vi "Fill Slider Values.vi"(10 "LBCB Number":T3, 11 "DofType":T2) -> (2 "Silder Values":T1(array[cluster]))   [LabVIEW 2009]
uses:
  Data Access Objects/Metadata/LBCB Number.ctl
  Data Access Objects/Limits/DofTypes.ctl
  Data Access Objects/Metadata/Persistant DAO Actions.ctl
  Global Data/Dataset Type.ctl
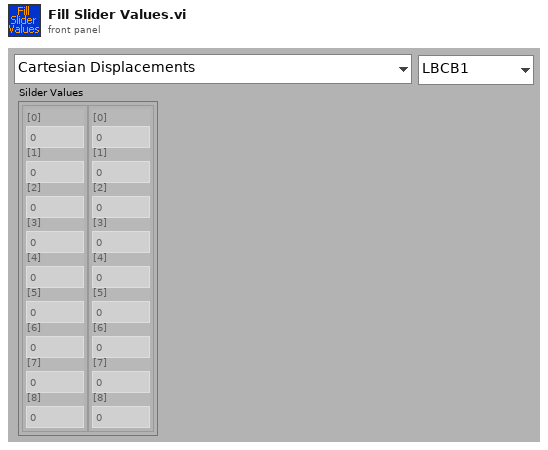
[diagram p1: front panel]
types:
  T1 = cluster{"[0]":dbl, "[1]":dbl, "[2]":dbl, "[3]":dbl, "[4]":dbl, "[5]":dbl, "[6]":dbl, "[7]":dbl, "[8]":dbl}[]
  T2 = typedef "DofTypes.ctl" = enum16{"Cartesian Displacements", "Cartesian Forces & Moments", "Actuator Displacements", "Actuator Forces", "Cartesian Increments", "Actuator Increments"}
  T3 = typedef "LBCB Number.ctl" = enum16{"LBCB1", "LBCB2"}
  T4 = typedef "Dataset Type.ctl" = enum16{"LVDT", "Load Cell", "Actuator Command", "Servo Error", "Displacement Command", "Displacement", "Force"}
  T5 = typedef "Persistant DAO Actions.ctl" = enum16{"Init", "Get", "Set", "Load", "Save"}
  T6 = typedef "Dataset Source.ctl" = enum16{"LBCB 1", "LBCB 2", "Combined", "External Sensors"}
  T7 = typedef "Dataset Transaction Id.ctl" = cluster{"Dataset Source":T6, "Dataset Type":T4, "Hold":T8, "Volts":T8, "Tag":string}
  T8 = typedef "Yes No Button.ctl" = bool
  T9 = typedef "Actuator Matrix.ctl" = cluster{"Lower":T10, "Upper":T10}
  T10 = typedef "Actuator Point.ctl" = cluster{"X1":dbl, "X2":dbl, "Y1":dbl, "Z1":dbl, "Z2":dbl, "Z3":dbl}
  T11 = typedef "Cartesian Point.ctl" = cluster{"Dx":dbl, "Dy":dbl, "Dz":dbl, "Rx":dbl, "Ry":dbl, "Rz":dbl}
  T12 = typedef "Cartesian Matrix.ctl" = cluster{"Lower":T11, "Upper":T11}
  T13 = typedef "Act & Cart Commands.ctl" = cluster{"Act Cmd":dbl[], "Cart Cmd":dbl[]}
  T14 = typedef "Limit Matrix.ctl" = dbl[][]
  T15 = cluster{"[0]":dbl, "[1]":dbl, "[2]":dbl, "[3]":dbl, "[4]":dbl, "[5]":dbl, "[6]":dbl, "[7]":dbl, "[8]":dbl}[][]
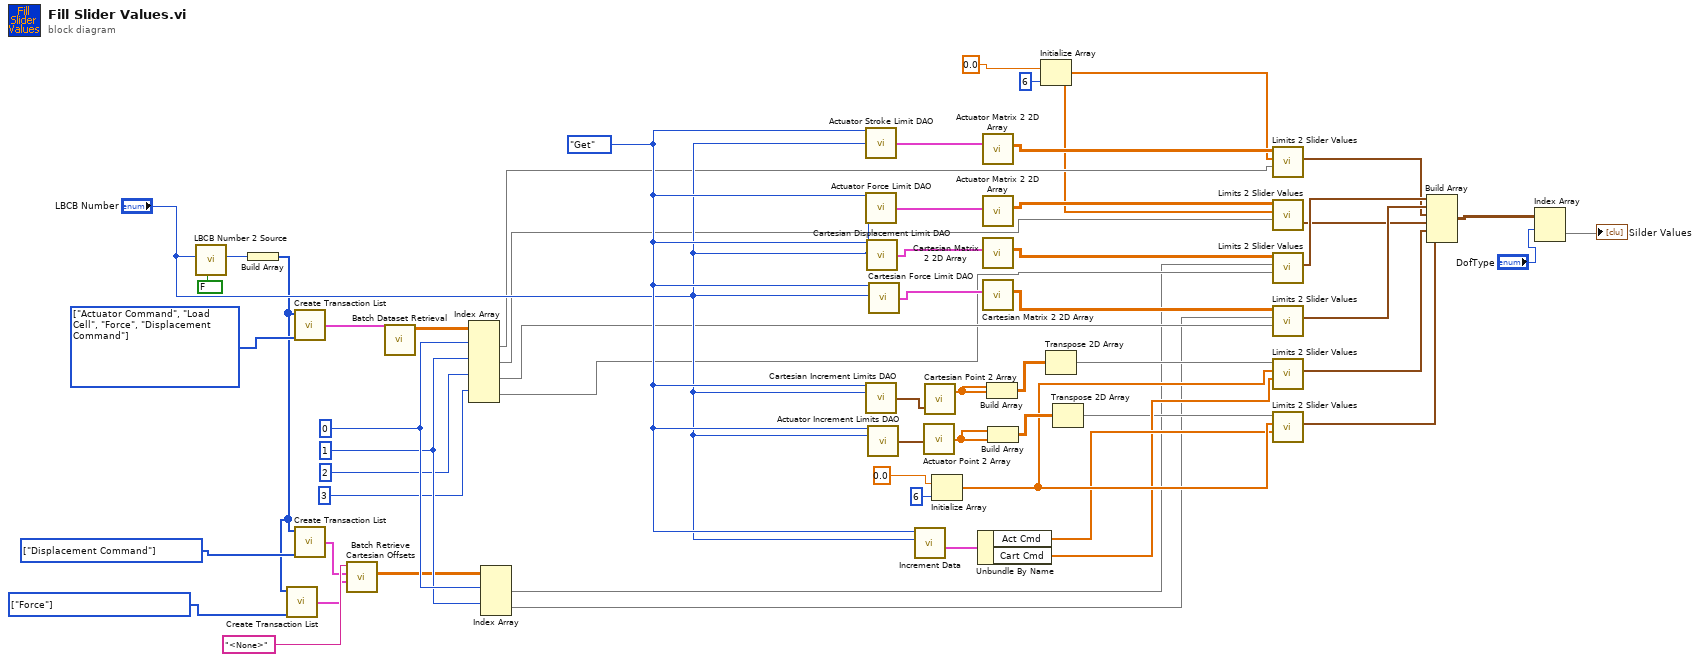
[diagram p0: block diagram]
diagram:
  w9 = T4[] [enum."Force"] items=["LVDT", "Load Cell", "Actuator Command", "Servo Error", "Displacement Command", "Displacement", "Force"] ("Types")
  w10 = T4[] [enum."Displacement Command"] items=["LVDT", "Load Cell", "Actuator Command", "Servo Error", "Displacement Command", "Displacement", "Force"] ("Types")
  w16 = 1 ("index")
  w17 = 0 ("index (row)")
  w26 = T4[] [enum."Actuator Command", enum."Load Cell", enum."Force", enum."Displacement Command"] items=["LVDT", "Load Cell", "Actuator Command", "Servo Error", "Displacement Command", "Displacement", "Force"] ("Types")
  w34 = Persistant_DAO_Actions."Get" ("Actuator Stroke Limit Actions")
  n1 = call "LBCB Number 2 Source.vi"("Combined"=FALSE, "LBCB Number"="LBCB Number") -> ("Dataset Source"=w25:T6)  [unwired: 9 in]
  n2 = Build Array(w25) -> (w8:T6[])
  n3 = call "Create Transaction List.vi"("Types"=w9, "Sources"=w8) -> ("Transactions"=w5:T7[])  [unwired: 2 in]
  n4 = call "Create Transaction List.vi"("Types"=w26, "Sources"=w8) -> ("Transactions"=w23:T7[])  [unwired: 2 in]
  n5 = call "Create Transaction List.vi"("Types"=w10, "Sources"=w8) -> ("Transactions"=w6:T7[])  [unwired: 2 in]
  n6 = call "Batch Retrieve Cartesian Offsets.vi"("Force Offsets"=w5, "Displacement Offsets"=w6, "Force Tag"="<None>") -> ("Offsets"=w4:dbl[][])  [unwired: 5 in, 1 out]
  n7 = call "Batch Dataset Retrieval.vi"("Transactions"=w23) -> ("Data"=w22:dbl[][])  [unwired: 9 in, 1 out]
  n8 = Index Array(array=w22, index (row) #1=w17, index (row) #2=w16, index (row) #3=2 ("index"), index (row) #4=3 ("index")) -> (element #1=w21:dbl[], element #2=w20:dbl[], element #3=w19:dbl[], element #4=w18:dbl[])  [unwired: 4 in]
  n9 = Index Array(array=w4, index (row) #1=w17, index (row) #2=w16) -> (element #1=w3:dbl[], element #2=w2:dbl[])  [unwired: 2 in]
  n10 = call "Actuator Stroke Limit DAO.vi"("Actuator Stroke Limit Actions"=w34, "ID"="LBCB Number") -> ("Actuator Stroke Limits Out"=w58:T9)  [unwired: 11 in, 2 out]
  n11 = call "Actuator Force Limit DAO.vi"("Actuator Force Limit Actions"=w34, "ID"="LBCB Number") -> ("Actuator Force Limits Out"=w57:T9)  [unwired: 11 in, 2 out]
  n12 = call "Cartesian Increment Limits DAO.vi"("Actions"=w34, "LBCB Number"="LBCB Number") -> ("Inc Limits Out"=w43:T11)  [unwired: 11 in, 2 out]
  n13 = call "Cartesian Displacement Limit DAO.vi"("Cartesian Displacement Limit Actions"=w34, "ID"="LBCB Number") -> ("Cartesian Displacement Out"=w56:T12)  [unwired: 11 in, 2 out]
  n14 = call "Actuator Increment Limits DAO.vi"("Actions"=w34, "LBCB Number"="LBCB Number") -> ("Inc Limits Out"=w42:T10)  [unwired: 11 in, 2 out]
  n15 = call "Cartesian Force Limit DAO.vi"("Cartesian Force Limit Actions"=w34, "ID"="LBCB Number") -> ("Cartesian Force Limit Out"=w55:T12)  [unwired: 11 in, 2 out]
  n16 = call "Increment Data.vi"("LBCB Number"="LBCB Number", "DAO Actions"=w34) -> ("Increments Out"=w33:T13)  [unwired: 8 in, 1 out]
  n17 = call "Actuator Point 2 Array.vi"("Actuator Point"=w42) -> ("Array"=w40:dbl[])
  n18 = call "Cartesian Point 2 Array.vi"("Cart Disp"=w43) -> ("Array"=w41:dbl[])  [unwired: 2 in]
  n19 = Initialize Array(0.0 ("element"), 6 ("dimension size")) -> (w35:dbl[])
  n20 = Unbundle By Name(w33) -> ("Act Cmd"=w32:dbl[], "Cart Cmd"=w31:dbl[])
  n21 = call "Actuator Matrix 2 2D Array.vi"("Matrix In"=w58) -> ("Matrix Out"=w54:T14)  [unwired: 10 in]
  n22 = call "Actuator Matrix 2 2D Array.vi"("Matrix In"=w57) -> ("Matrix Out"=w53:T14)  [unwired: 10 in]
  n23 = call "Cartesian Matrix 2 2D Array.vi"("Matrix In"=w56) -> ("Matrix Out"=w52:T14)  [unwired: 10 in]
  n24 = call "Cartesian Matrix 2 2D Array.vi"("Matrix In"=w55) -> ("Matrix Out"=w51:T14)  [unwired: 10 in]
  n25 = Build Array(w41, w41) -> (w39:dbl[][])
  n26 = Build Array(w40, w40) -> (w38:dbl[][])
  n27 = Initialize Array(0.0, 6 ("dimension size")) -> (w11:dbl[])
  n28 = Transpose 2D Array(2D array=w39) -> (transposed array=w28:dbl[][])
  n29 = Transpose 2D Array(2D array=w38) -> (transposed array=w27:dbl[][])
  n30 = call "Limits 2 Slider Values.vi"("Actual"=w21, "Offsets"=w11, "Limits"=w54) -> ("Values"=w48:T1)  [unwired: 8 in]
  n31 = call "Limits 2 Slider Values.vi"("Actual"=w20, "Offsets"=w11, "Limits"=w53) -> ("Values"=w47:T1)  [unwired: 8 in]
  n32 = call "Limits 2 Slider Values.vi"("Actual"=w18, "Offsets"=w3, "Limits"=w52) -> ("Values"=w50:T1)  [unwired: 8 in]
  n33 = call "Limits 2 Slider Values.vi"("Actual"=w19, "Offsets"=w2, "Limits"=w51) -> ("Values"=w49:T1)  [unwired: 8 in]
  n34 = call "Limits 2 Slider Values.vi"("Actual"=w31, "Offsets"=w35, "Limits"=w28) -> ("Values"=w30:T1)  [unwired: 8 in]
  n35 = call "Limits 2 Slider Values.vi"("Actual"=w32, "Offsets"=w35, "Limits"=w27) -> ("Values"=w29:T1)  [unwired: 8 in]
  n36 = Build Array(w50, w49, w48, w47, w30, w29) -> (w46:T15)
  n37 = Index Array(array=w46, index (row)="DofType") -> (element=→"Silder Values":T1)  [unwired: 1 in]
